vi "Distance and Stuff.vi"() -> ()   [LabVIEW 2015]
panel:
  out "Maxsonar distance":dbl
  out "Infrared distance":dbl
  out "Ultarsonic Yaw":dbl
  out "Lidar Depth Value":dbl
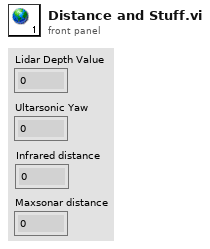
[diagram p1: front panel]
diagram:
